vi "List Roots.vi"(8 "Error In":errorcluster, 11 "Tree":T1) -> (0 "Error Out":errorcluster, 1 "Roots Names":string[](array[string]), 3 "Tree":T1, 5 "Roots IDs":string[](array[string]))   [LabVIEW 2020, in "NI_VIAnCFGDataStructure.lvlib" / "Tree.lvclass"]
doc: "List the Trees that have no Parent ID specified.\n\nThe list order is random."
uses:
  <vilib>/addons/analyzer/VIAnCFGDataStructure/Tree Manager/Tree.lvclass
  <vilib>/addons/analyzer/VIAnCFGDataStructure/Tree Manager/Typedefs/Session Handle.ctl
  <vilib>/addons/analyzer/VIAnCFGDataStructure/Tree Manager/Tree.lvclass/Tree.ctl
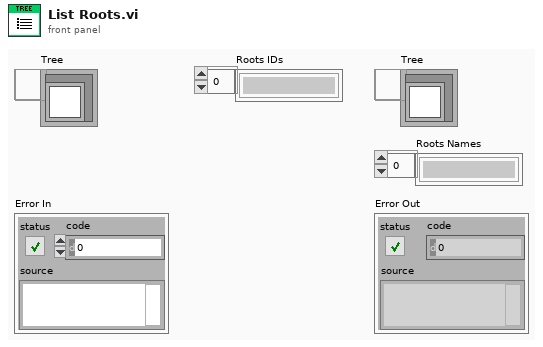
[diagram p1: front panel]
types:
  T1 = typedef "NI_VIAnCFGDataStructure.lvlib/Tree.lvclass/Session Handle.ctl" = refnum<data-value>
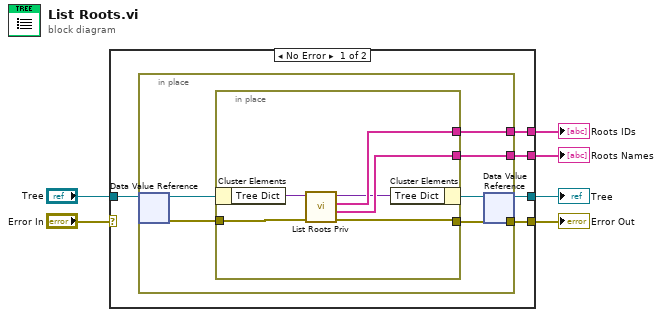
[diagram p0: block diagram]
diagram:
  n1 = case shown="No Error" "Error In" {
    selector: "Error In" -> [_ w24]
    tunnel: "Tree" -> [w11 w25]
    tunnel: [w10 w25] -> w5
    tunnel: [w9 w24] -> w3
    tunnel: [w8 _] -> w2
    tunnel: [w7 _] -> w1
    frame No Error {
      n2 = in-place {
        in-place-border: [w16] -> w9
        in-place-border: [w13] -> w8
        in-place-border: [w12] -> w7
        n3 = in-place-dvr #1(w11) -> (w17:refnum<class "Tree.lvclass">, w14:errorcluster)
        n4 = in-place {
          in-place-border: [w18] -> w16
          in-place-border: w14 -> [w22]
          in-place-border: [w21] -> w13
          in-place-border: [w20] -> w12
          n5 = in-place-cluster #2(w17) -> ("Tree Dict"=w23:variant)
          n6 = call <vilib>:"List Roots Priv.vi"("error in"=w22, "Tree Dict"=w23) -> ("error out"=w18:errorcluster, "Root Names"=w20:string[], "Root IDs"=w21:string[], "Tree Dict"=w19:variant)  [unwired: 6 in]
          n7 = in-place-cluster #2("Tree Dict"=w19) -> (w15:refnum<class "Tree.lvclass">)
        }
        n8 = in-place-dvr #1(w15) -> (w10:T1)  [unwired: 1 out]
      }
    }
    frame Error {
    }
  }
  "Tree" <- w5
  "Error Out" <- w3
  "Roots IDs" <- w2
  "Roots Names" <- w1
